vi "Calcfactor.vi"(1 "Preamp Sensitivity":T2(ring)=enum."100nA/V", 2 "Configuration 2":T1(ring), 3 "Multiply Data?":bool, 4 "Lockin resource":refnum<visa-resource-name>="COM12") -> (0 "Multiplication Factor":dbl)   [LabVIEW 2013]
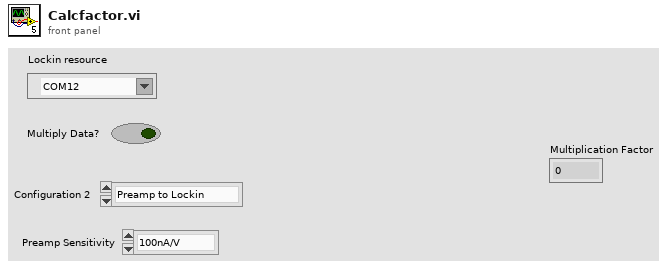
[diagram p1: front panel]
types:
  T1 = enum16{"Preamp to Lockin", "Preamp", "Lockin current", "Lockin Voltage", ""}
  T2 = enum16{"1pA/V", "2pA/V", "5pA/V", "10pA/V", "20pA/V", "50pA/V", "100pA/V", "200pA/V", "500pA/V", "1nA/V", "2nA/V", "5nA/V", "10nA/V", "20nA/V", "50nA/V", "100nA/V", "200nA/V", "500nA/V", "1uA/V", "2uA/V", "5uA/V", "10uA/V", "20uA/V", "50uA/V", "100uA/V", "200uA/V", "500uA/V", "1mA/V"}
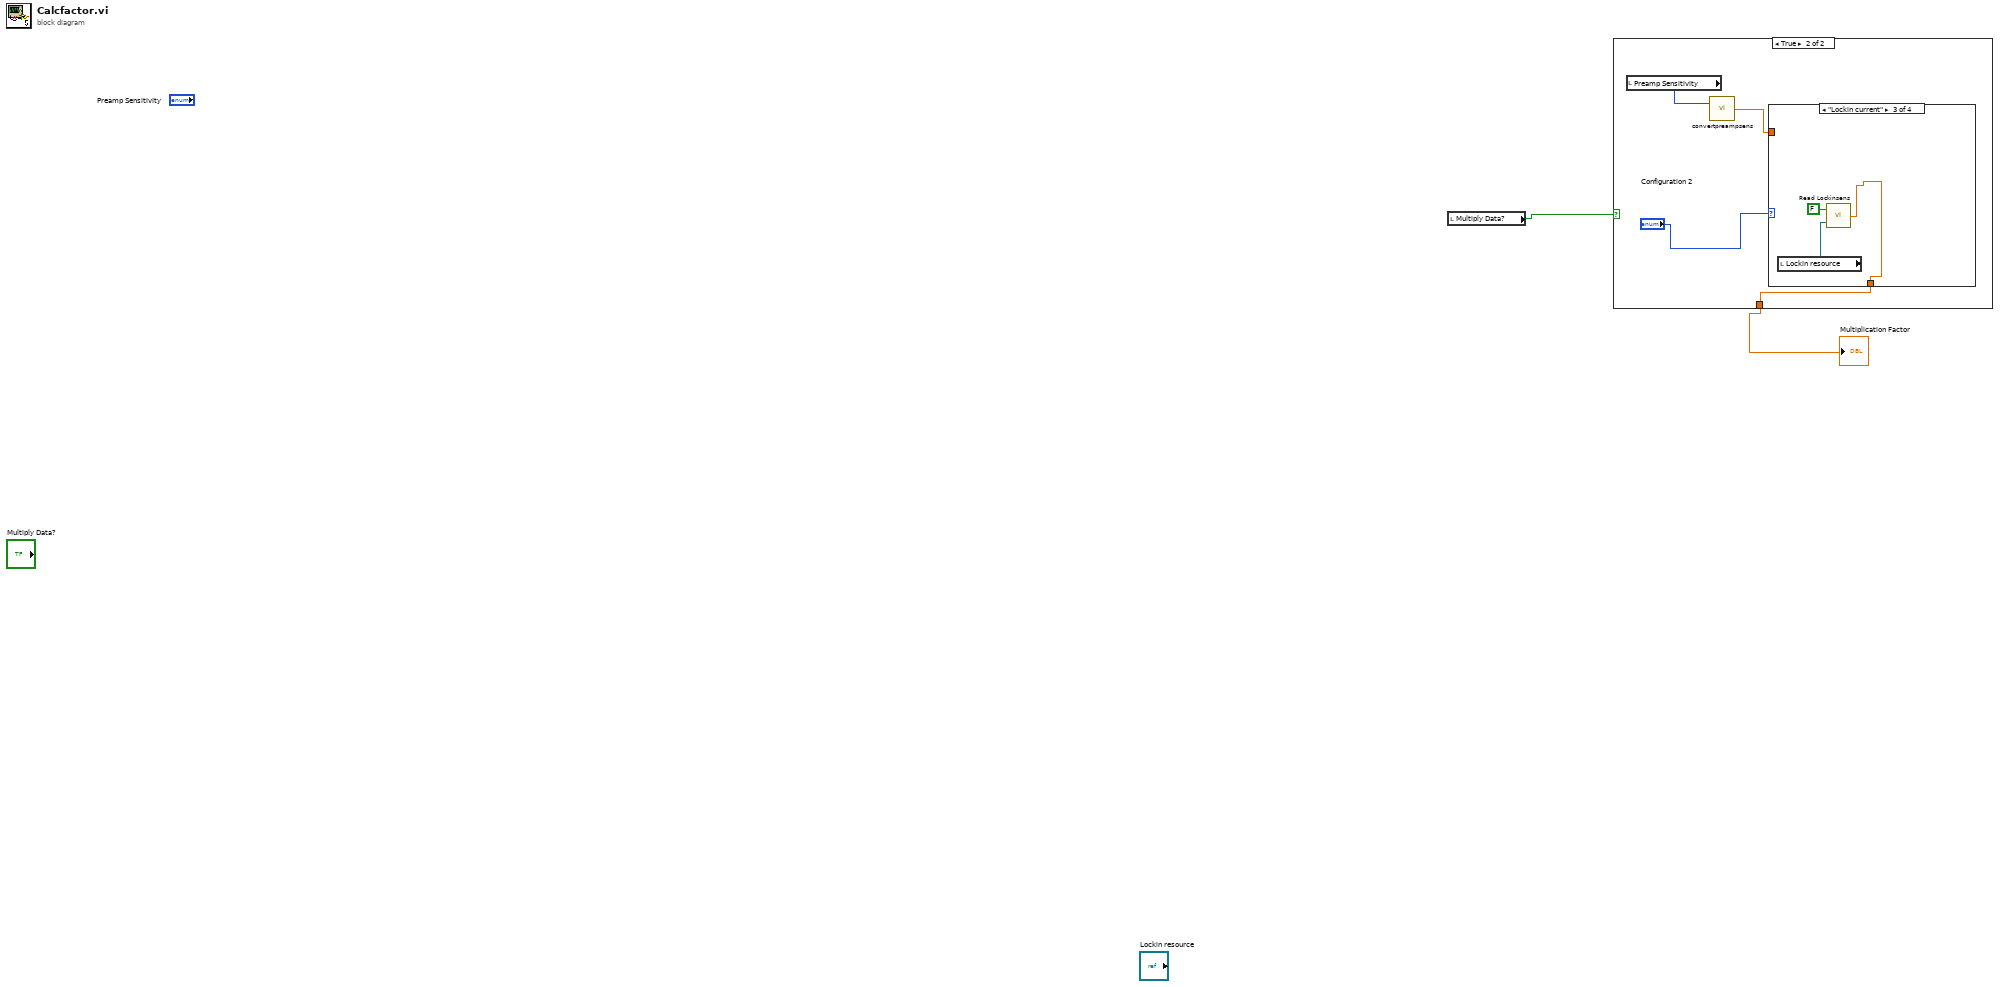
[diagram p0: block diagram]
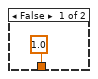
[diagram p2: hidden frame]
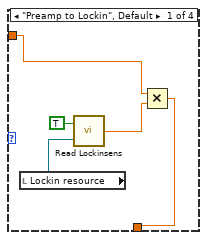
[diagram p3: hidden frame]
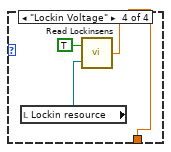
[diagram p5: hidden frame]
diagram:
  n1 = local read "Multiply Data?"() -> (w2:bool)
  n2 = case shown="True" w2 {
    tunnel: [1.0 ("Sensitivity") w7] -> w1
    frame False {
    }
    frame True {
      n3 = local read "Preamp Sensitivity"() -> (w6:T2)
      n4 = call "convertpreampsens.vi"("Preamp Sensitivity"=w6) -> ("Sensitivity"=w5:dbl)  [unwired: 1 in]
      n5 = case shown="\"Lockin current\"" "Configuration 2" {
        tunnel: [w10 w13 w14 w17] -> w7
        tunnel: w5 -> [w8 w13 _ _]
        frame "Preamp to Lockin", Default {
          n6 = local read "Lockin resource"() -> (w12:refnum<visa-resource-name>)
          n7 = call "Read Lockinsens.vi"("VISA resource name"=w12, "Voltage(T) Current(F)"=TRUE) -> ("Sensitivity"=w11:dbl)
          n8 = Multiply(x=w8, y=w11) -> (x*y=w10:dbl)
        }
        frame "Preamp" {
        }
        frame "Lockin current" {
          n9 = local read "Lockin resource"() -> (w16:refnum<visa-resource-name>)
          n10 = call "Read Lockinsens.vi"("VISA resource name"=w16, "Voltage(T) Current(F)"=FALSE) -> ("Sensitivity"=w14:dbl)
        }
        frame "Lockin Voltage" {
          n11 = local read "Lockin resource"() -> (w19:refnum<visa-resource-name>)
          n12 = call "Read Lockinsens.vi"("VISA resource name"=w19, "Voltage(T) Current(F)"=TRUE) -> ("Sensitivity"=w17:dbl)
        }
      }
    }
  }
  "Multiplication Factor" <- w1
